vi "Read Sub panel msg.vi"(8 "error in (no error)":errorcluster, 11 "Mensaje Actor in":refnum<class "Mensaje Actor.lvclass">) -> (0 "error out":errorcluster, 2 "Sub panel msg":refnum<vi>, 3 "Mensaje Actor out":refnum<class "Mensaje Actor.lvclass">)   [LabVIEW 2019, in "Mensaje Actor.lvlib" / "Mensaje Actor.lvclass"]
uses:
  Mensaje Actor.lvclass
  Mensaje Actor.lvclass/Mensaje Actor.ctl
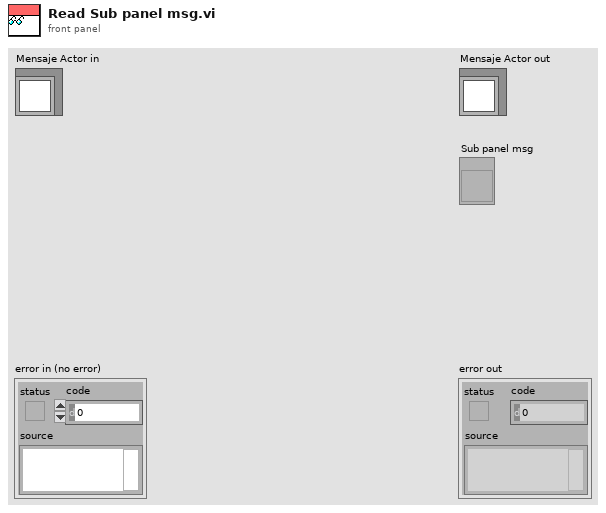
[diagram p1: front panel]
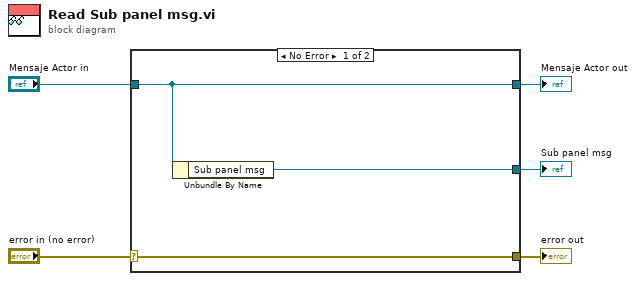
[diagram p0: block diagram]
diagram:
  n1 = case shown="No Error" "error in (no error)" {
    selector: "error in (no error)" -> [w8 w9]
    tunnel: [w8 w9] -> w4
    tunnel: [w7 w10] -> w2
    tunnel: "Mensaje Actor in" -> [w7 w10]
    tunnel: [w6 _] -> w1
    frame No Error {
      n2 = Unbundle By Name(w7) -> ("Sub panel msg"=w6:refnum<vi>)
    }
    frame Error {
    }
  }
  "error out" <- w4
  "Mensaje Actor out" <- w2
  "Sub panel msg" <- w1
